vi "Main GNSS-Gmap.vi"() -> ()   [LabVIEW 2019]
uses:
  C:/Users/WEGO/Documents/GitHub/Ycar/LabVIEW/Gmap/dll/GMap.NET.WindowsForms.dll
  Gmap/dll/GMap.NET.WindowsForms.dll
  Ctrl/ublox-ui_main.ctl
  Ctrl/gnss_config-2.ctl
  Ctrl/cmd_RW.ctl
  Ctrl/cmd_ini-RW.ctl
  Ctrl/cmd_common.ctl
  Ctrl/comm-ini-rw-close.ctl
  Gmap/gmap_fgv-cmd.ctl
  Gmap/marker_info.ctl
panel:
  in  "main tap":enum32{"Main", "설정"}(tab)
  out "Ntrip conn":bool
  out "Sea Level":dbl
  out "N of Satellites":i32
  out "GNSS time":string
  in  "tm data reset":bool
  in  "gnss mode check":bool
  in  "GMapControl":refnum<k24>(container)
  out "TM graph":T1(graph)=[{"TM array"=[{"Y(E)"=195478.83340938148, "X(N)"=532749.6315443226}, {"Y(E)"=195478.83340938148, "X(N)"=532749.6315443226}, {"Y(E)"=195478.83340938148, "X(N)"=532749.6315443226}, {"Y(E)"=195478.83340938148, "X(N)"=532749.6315443226}, {"Y(E)"=195478.83340938148, "X(N)"=532749.6315443226}, {"Y(E)"=195478.83340938148, "X(N)"=532749.6315443226}, {"Y(E)"=195478.83340938148, "X(N)"=532749.6315443226}, {"Y(E)"=195478.83340938148, "X(N)"=532749.6315443226}, {"Y(E)"=195478.83340938148, "X(N)"=532749.6315443226}, {"Y(E)"=195478.83340938148, "X(N)"=532749.6315443226}, {"Y(E)"=195478.80387262133, "X(N)"=532749.5945652778}, {"Y(E)"=195478.80387262133, "X(N)"=532749.5945652778}, {"Y(E)"=195478.80387262133, "X(N)"=532749.5945652778}, {"Y(E)"=195478.80387262133, "X(N)"=532749.5945652778}, {"Y(E)"=195478.80387262133, "X(N)"=532749.5945652778}, {"Y(E)"=195478.80387262133, "X(N)"=532749.5945652778}, {"Y(E)"=195478.80387262133, "X(N)"=532749.5945652778}, {"Y(E)"=195478.80387262133, "X(N)"=532749.5945652778}, {"Y(E)"=195478.80387262133, "X(N)"=532749.5945652778}, {"Y(E)"=195478.80387262133, "X(N)"=532749.5945652778}, {"Y(E)"=195478.80387262133, "X(N)"=532749.5945652778}, {"Y(E)"=195478.80387262133, "X(N)"=532749.5945652778}, {"Y(E)"=195478.80387262133, "X(N)"=532749.5945652778}, {"Y(E)"=195478.86283602339, "X(N)"=532749.4650507653}, {"Y(E)"=195478.86283602339, "X(N)"=532749.4650507653}, {"Y(E)"=195478.86283602339, "X(N)"=532749.4650507653}, {"Y(E)"=195478.86283602339, "X(N)"=532749.4650507653}, {"Y(E)"=195478.86283602339, "X(N)"=532749.4650507653}, {"Y(E)"=195478.86283602339, "X(N)"=532749.4650507653}, {"Y(E)"=195478.86283602339, "X(N)"=532749.4650507653}, {"Y(E)"=195478.86283602339, "X(N)"=532749.4650507653}, {"Y(E)"=195478.86283602339, "X(N)"=532749.4650507653}, {"Y(E)"=195478.86283602339, "X(N)"=532749.4650507653}, {"Y(E)"=195478.86283602339, "X(N)"=532749.4650507653}, {"Y(E)"=195478.86283602339, "X(N)"=532749.4650507653}, {"Y(E)"=195478.86283602339, "X(N)"=532749.4650507653}, {"Y(E)"=195478.8185809412, "X(N)"=532749.5020697443}, {"Y(E)"=195478.8185809412, "X(N)"=532749.5020697443}, {"Y(E)"=195478.8185809412, "X(N)"=532749.5020697443}, {"Y(E)"=195478.8185809412, "X(N)"=532749.5020697443}, {"Y(E)"=195478.8185809412, "X(N)"=532749.5020697443}, {"Y(E)"=195478.8185809412, "X(N)"=532749.5020697443}, {"Y(E)"=195478.8185809412, "X(N)"=532749.5020697443}, {"Y(E)"=195478.8185809412, "X(N)"=532749.5020697443}, {"Y(E)"=195478.8185809412, "X(N)"=532749.5020697443}, {"Y(E)"=195478.8185809412, "X(N)"=532749.5020697443}, {"Y(E)"=195478.8185809412, "X(N)"=532749.5020697443}, {"Y(E)"=195478.8185809412, "X(N)"=532749.5020697443}, {"Y(E)"=195478.8185809412, "X(N)"=532749.5020697443}, {"Y(E)"=195478.8333493192, "X(N)"=532749.5205592669}, {"Y(E)"=195478.8333493192, "X(N)"=532749.5205592669}, {"Y(E)"=195478.8333493192, "X(N)"=532749.5205592669}, {"Y(E)"=195478.8333493192, "X(N)"=532749.5205592669}, {"Y(E)"=195478.8333493192, "X(N)"=532749.5205592669}, {"Y(E)"=195478.8333493192, "X(N)"=532749.5205592669}, {"Y(E)"=195478.8333493192, "X(N)"=532749.5205592669}, {"Y(E)"=195478.8333493192, "X(N)"=532749.5205592669}, {"Y(E)"=195478.8333493192, "X(N)"=532749.5205592669}, {"Y(E)"=195478.8333493192, "X(N)"=532749.5205592669}, {"Y(E)"=195478.8333493192, "X(N)"=532749.5205592669}, {"Y(E)"=195478.8333493192, "X(N)"=532749.5205592669}, {"Y(E)"=195478.81854089958, "X(N)"=532749.4280797082}, {"Y(E)"=195478.81854089958, "X(N)"=532749.4280797082}, {"Y(E)"=195478.81854089958, "X(N)"=532749.4280797082}, {"Y(E)"=195478.81854089958, "X(N)"=532749.4280797082}, {"Y(E)"=195478.81854089958, "X(N)"=532749.4280797082}, {"Y(E)"=195478.81854089958, "X(N)"=532749.4280797082}, {"Y(E)"=195478.81854089958, "X(N)"=532749.4280797082}, {"Y(E)"=195478.81854089958, "X(N)"=532749.4280797082}, {"Y(E)"=195478.81854089958, "X(N)"=532749.4280797082}, {"Y(E)"=195478.81854089958, "X(N)"=532749.4280797082}, {"Y(E)"=195478.81854089958, "X(N)"=532749.4280797082}, {"Y(E)"=195478.81854089958, "X(N)"=532749.4280797082}, {"Y(E)"=195478.81854089958, "X(N)"=532749.4280797082}, {"Y(E)"=195478.8332592258, "X(N)"=532749.3540816847}, {"Y(E)"=195478.8332592258, "X(N)"=532749.3540816847}, {"Y(E)"=195478.8332592258, "X(N)"=532749.3540816847}, {"Y(E)"=195478.8332592258, "X(N)"=532749.3540816847}, {"Y(E)"=195478.8332592258, "X(N)"=532749.3540816847}, {"Y(E)"=195478.8332592258, "X(N)"=532749.3540816847}, {"Y(E)"=195478.8332592258, "X(N)"=532749.3540816847}, {"Y(E)"=195478.8332592258, "X(N)"=532749.3540816847}, {"Y(E)"=195478.8332592258, "X(N)"=532749.3540816847}, {"Y(E)"=195478.8332592258, "X(N)"=532749.3540816847}, {"Y(E)"=195478.8332592258, "X(N)"=532749.3540816847}, {"Y(E)"=195478.8332592258, "X(N)"=532749.3540816847}, {"Y(E)"=195478.8332592258, "X(N)"=532749.3540816847}, {"Y(E)"=195478.61200383154, "X(N)"=532749.5761715989}, {"Y(E)"=195478.61200383154, "X(N)"=532749.5761715989}, {"Y(E)"=195478.61200383154, "X(N)"=532749.5761715989}, {"Y(E)"=195478.61200383154, "X(N)"=532749.5761715989}, {"Y(E)"=195478.61200383154, "X(N)"=532749.5761715989}, {"Y(E)"=195478.61200383154, "X(N)"=532749.5761715989}, {"Y(E)"=195478.61200383154, "X(N)"=532749.5761715989}, {"Y(E)"=195478.61200383154, "X(N)"=532749.5761715989}, {"Y(E)"=195478.61200383154, "X(N)"=532749.5761715989}, {"Y(E)"=195478.61200383154, "X(N)"=532749.5761715989}, {"Y(E)"=195478.61200383154, "X(N)"=532749.5761715989}, {"Y(E)"=195478.61200383154, "X(N)"=532749.5761715989}, {"Y(E)"=195478.61200383154, "X(N)"=532749.5761715989}, {"Y(E)"=195478.61197379892, "X(N)"=532749.5206790727}, {"Y(E)"=195478.61197379892, "X(N)"=532749.5206790727}, {"Y(E)"=195478.61197379892, "X(N)"=532749.5206790727}, {"Y(E)"=195478.61197379892, "X(N)"=532749.5206790727}, {"Y(E)"=195478.61197379892, "X(N)"=532749.5206790727}, {"Y(E)"=195478.61197379892, "X(N)"=532749.5206790727}, {"Y(E)"=195478.61197379892, "X(N)"=532749.5206790727}, {"Y(E)"=195478.61197379892, "X(N)"=532749.5206790727}, {"Y(E)"=195478.61197379892, "X(N)"=532749.5206790727}, {"Y(E)"=195478.61197379892, "X(N)"=532749.5206790727}, {"Y(E)"=195478.61197379892, "X(N)"=532749.5206790727}, {"Y(E)"=195478.61197379892, "X(N)"=532749.5206790727}, {"Y(E)"=195478.61197379892, "X(N)"=532749.5206790727}, {"Y(E)"=195478.64144048005, "X(N)"=532749.4281755526}, {"Y(E)"=195478.64144048005, "X(N)"=532749.4281755526}, {"Y(E)"=195478.64144048005, "X(N)"=532749.4281755526}, {"Y(E)"=195478.64144048005, "X(N)"=532749.4281755526}, {"Y(E)"=195478.64144048005, "X(N)"=532749.4281755526}, {"Y(E)"=195478.64144048005, "X(N)"=532749.4281755526}, {"Y(E)"=195478.64144048005, "X(N)"=532749.4281755526}, {"Y(E)"=195478.64144048005, "X(N)"=532749.4281755526}, {"Y(E)"=195478.64144048005, "X(N)"=532749.4281755526}, {"Y(E)"=195478.64144048005, "X(N)"=532749.4281755526}, {"Y(E)"=195478.64144048005, "X(N)"=532749.4281755526}, {"Y(E)"=195478.64144048005, "X(N)"=532749.4281755526}, {"Y(E)"=195478.64144048005, "X(N)"=532749.4281755526}, {"Y(E)"=195478.56754852948, "X(N)"=532749.2432403986}, {"Y(E)"=195478.56754852948, "X(N)"=532749.2432403986}, {"Y(E)"=195478.56754852948, "X(N)"=532749.2432403986}, {"Y(E)"=195478.56754852948, "X(N)"=532749.2432403986}, {"Y(E)"=195478.56754852948, "X(N)"=532749.2432403986}, {"Y(E)"=195478.56754852948, "X(N)"=532749.2432403986}, {"Y(E)"=195478.56754852948, "X(N)"=532749.2432403986}, {"Y(E)"=195478.56754852948, "X(N)"=532749.2432403986}, {"Y(E)"=195478.56754852948, "X(N)"=532749.2432403986}, {"Y(E)"=195478.56754852948, "X(N)"=532749.2432403986}, {"Y(E)"=195478.56754852948, "X(N)"=532749.2432403986}, {"Y(E)"=195478.56754852948, "X(N)"=532749.2432403986}, {"Y(E)"=195478.56754852948, "X(N)"=532749.2432403986}, {"Y(E)"=195478.5822568451, "X(N)"=532749.1507448669}, {"Y(E)"=195478.5822568451, "X(N)"=532749.1507448669}, {"Y(E)"=195478.5822568451, "X(N)"=532749.1507448669}, {"Y(E)"=195478.5822568451, "X(N)"=532749.1507448669}, {"Y(E)"=195478.5822568451, "X(N)"=532749.1507448669}, {"Y(E)"=195478.5822568451, "X(N)"=532749.1507448669}, {"Y(E)"=195478.5822568451, "X(N)"=532749.1507448669}, {"Y(E)"=195478.5822568451, "X(N)"=532749.1507448669}, {"Y(E)"=195478.5822568451, "X(N)"=532749.1507448669}, {"Y(E)"=195478.5822568451, "X(N)"=532749.1507448669}, {"Y(E)"=195478.5822568451, "X(N)"=532749.1507448669}, {"Y(E)"=195478.5822568451, "X(N)"=532749.1507448669}, {"Y(E)"=195478.5822568451, "X(N)"=532749.1507448669}, {"Y(E)"=195478.3755095352, "X(N)"=532748.9103890732}, {"Y(E)"=195478.3755095352, "X(N)"=532748.9103890732}, {"Y(E)"=195478.3755095352, "X(N)"=532748.9103890732}, {"Y(E)"=195478.3755095352, "X(N)"=532748.9103890732}, {"Y(E)"=195478.3755095352, "X(N)"=532748.9103890732}, {"Y(E)"=195478.3755095352, "X(N)"=532748.9103890732}, {"Y(E)"=195478.3755095352, "X(N)"=532748.9103890732}, {"Y(E)"=195478.3755095352, "X(N)"=532748.9103890732}, {"Y(E)"=195478.3755095352, "X(N)"=532748.9103890732}, {"Y(E)"=195478.3755095352, "X(N)"=532748.9103890732}, {"Y(E)"=195478.3755095352, "X(N)"=532748.9103890732}, {"Y(E)"=195478.3755095352, "X(N)"=532748.9103890732}, {"Y(E)"=195478.3755095352, "X(N)"=532748.9103890732}, {"Y(E)"=195478.37543945547, "X(N)"=532748.78090651}, {"Y(E)"=195478.37543945547, "X(N)"=532748.78090651}, {"Y(E)"=195478.37543945547, "X(N)"=532748.78090651}, {"Y(E)"=195478.37543945547, "X(N)"=532748.78090651}, {"Y(E)"=195478.37543945547, "X(N)"=532748.78090651}, {"Y(E)"=195478.37543945547, "X(N)"=532748.78090651}, {"Y(E)"=195478.37543945547, "X(N)"=532748.78090651}, {"Y(E)"=195478.37543945547, "X(N)"=532748.78090651}, {"Y(E)"=195478.37543945547, "X(N)"=532748.78090651}, {"Y(E)"=195478.37543945547, "X(N)"=532748.78090651}, {"Y(E)"=195478.37543945547, "X(N)"=532748.78090651}, {"Y(E)"=195478.37543945547, "X(N)"=532748.78090651}, {"Y(E)"=195478.5082848043, "X(N)"=532748.8178296402}, {"Y(E)"=195478.5082848043, "X(N)"=532748.8178296402}, {"Y(E)"=195478.5082848043, "X(N)"=532748.8178296402}, {"Y(E)"=195478.5082848043, "X(N)"=532748.8178296402}, {"Y(E)"=195478.5082848043, "X(N)"=532748.8178296402}, {"Y(E)"=195478.5082848043, "X(N)"=532748.8178296402}, {"Y(E)"=195478.5082848043, "X(N)"=532748.8178296402}, {"Y(E)"=195478.5082848043, "X(N)"=532748.8178296402}, {"Y(E)"=195478.5082848043, "X(N)"=532748.8178296402}, {"Y(E)"=195478.5082848043, "X(N)"=532748.8178296402}, {"Y(E)"=195478.5082848043, "X(N)"=532748.8178296402}, {"Y(E)"=195478.5082848043, "X(N)"=532748.8178296402}, {"Y(E)"=195478.5082848043, "X(N)"=532748.8178296402}, {"Y(E)"=195478.7001636224, "X(N)"=532748.8547208244}, {"Y(E)"=195478.7001636224, "X(N)"=532748.8547208244}, {"Y(E)"=195478.7001636224, "X(N)"=532748.8547208244}, {"Y(E)"=195478.7001636224, "X(N)"=532748.8547208244}, {"Y(E)"=195478.7001636224, "X(N)"=532748.8547208244}, {"Y(E)"=195478.7001636224, "X(N)"=532748.8547208244}, {"Y(E)"=195478.7001636224, "X(N)"=532748.8547208244}, {"Y(E)"=195478.7001636224, "X(N)"=532748.8547208244}, {"Y(E)"=195478.7001636224, "X(N)"=532748.8547208244}, {"Y(E)"=195478.7001636224, "X(N)"=532748.8547208244}]}, {"TM array"=[{"Y(E)"=195478.60442441847, "X(N)"=532749.6892681528}, {"Y(E)"=195478.63475492285, "X(N)"=532749.6883149784}, {"Y(E)"=195478.6649657266, "X(N)"=532749.6854592166}, {"Y(E)"=195478.69493760145, "X(N)"=532749.680712138}, {"Y(E)"=195478.72455226214, "X(N)"=532749.6740924771}, {"Y(E)"=195478.7536928331, "X(N)"=532749.6656263586}, {"Y(E)"=195478.7822443098, "X(N)"=532749.6553471944}, {"Y(E)"=195478.81009401265, "X(N)"=532749.6432955518}, {"Y(E)"=195478.83713203156, "X(N)"=532749.6295189931}, {"Y(E)"=195478.86325165984, "X(N)"=532749.6140718879}, {"Y(E)"=195478.88834981524, "X(N)"=532749.5970151991}, {"Y(E)"=195478.91232744683, "X(N)"=532749.5784162417}, {"Y(E)"=195478.93508992583, "X(N)"=532749.5583484169}, {"Y(E)"=195478.95654741913, "X(N)"=532749.5368909236}, {"Y(E)"=195478.97661524382, "X(N)"=532749.5141284446}, {"Y(E)"=195478.99521420136, "X(N)"=532749.490150813}, {"Y(E)"=195479.01227089018, "X(N)"=532749.4650526576}, {"Y(E)"=195479.02771799528, "X(N)"=532749.4389330294}, {"Y(E)"=195479.04149455403, "X(N)"=532749.4118950105}, {"Y(E)"=195479.0535461966, "X(N)"=532749.3840453076}, {"Y(E)"=195479.06382536073, "X(N)"=532749.3554938309}, {"Y(E)"=195479.0722914792, "X(N)"=532749.32635326}, {"Y(E)"=195479.07891114015, "X(N)"=532749.2967385993}, {"Y(E)"=195479.0836582188, "X(N)"=532749.2667667244}, {"Y(E)"=195479.08651398055, "X(N)"=532749.2365559207}, {"Y(E)"=195479.08746715504, "X(N)"=532749.2062254163}, {"Y(E)"=195479.08651398055, "X(N)"=532749.1758949119}, {"Y(E)"=195479.0836582188, "X(N)"=532749.1456841081}, {"Y(E)"=195479.07891114015, "X(N)"=532749.1157122332}, {"Y(E)"=195479.0722914792, "X(N)"=532749.0860975726}, {"Y(E)"=195479.06382536073, "X(N)"=532749.0569570017}, {"Y(E)"=195479.0535461966, "X(N)"=532749.0284055249}, {"Y(E)"=195479.04149455403, "X(N)"=532749.000555822}, {"Y(E)"=195479.02771799528, "X(N)"=532748.9735178031}, {"Y(E)"=195479.01227089018, "X(N)"=532748.9473981749}, {"Y(E)"=195478.99521420136, "X(N)"=532748.9223000195}, {"Y(E)"=195478.97661524382, "X(N)"=532748.898322388}, {"Y(E)"=195478.95654741913, "X(N)"=532748.8755599089}, {"Y(E)"=195478.93508992583, "X(N)"=532748.8541024156}, {"Y(E)"=195478.91232744683, "X(N)"=532748.8340345909}, {"Y(E)"=195478.88834981524, "X(N)"=532748.8154356334}, {"Y(E)"=195478.86325165984, "X(N)"=532748.7983789446}, {"Y(E)"=195478.83713203156, "X(N)"=532748.7829318395}, {"Y(E)"=195478.81009401265, "X(N)"=532748.7691552808}, {"Y(E)"=195478.7822443098, "X(N)"=532748.7571036381}, {"Y(E)"=195478.7536928331, "X(N)"=532748.746824474}, {"Y(E)"=195478.72455226214, "X(N)"=532748.7383583555}, {"Y(E)"=195478.69493760145, "X(N)"=532748.7317386946}, {"Y(E)"=195478.6649657266, "X(N)"=532748.726991616}, {"Y(E)"=195478.63475492285, "X(N)"=532748.7241358542}, {"Y(E)"=195478.60442441847, "X(N)"=532748.7231826797}, {"Y(E)"=195478.5740939141, "X(N)"=532748.7241358542}, {"Y(E)"=195478.54388311034, "X(N)"=532748.726991616}, {"Y(E)"=195478.5139112355, "X(N)"=532748.7317386946}, {"Y(E)"=195478.4842965748, "X(N)"=532748.7383583555}, {"Y(E)"=195478.45515600385, "X(N)"=532748.746824474}, {"Y(E)"=195478.42660452714, "X(N)"=532748.7571036381}, {"Y(E)"=195478.3987548243, "X(N)"=532748.7691552808}, {"Y(E)"=195478.37171680538, "X(N)"=532748.7829318395}, {"Y(E)"=195478.3455971771, "X(N)"=532748.7983789446}, {"Y(E)"=195478.3204990217, "X(N)"=532748.8154356334}, {"Y(E)"=195478.29652139012, "X(N)"=532748.8340345909}, {"Y(E)"=195478.27375891112, "X(N)"=532748.8541024156}, {"Y(E)"=195478.25230141782, "X(N)"=532748.8755599089}, {"Y(E)"=195478.23223359312, "X(N)"=532748.898322388}, {"Y(E)"=195478.21363463558, "X(N)"=532748.9223000195}, {"Y(E)"=195478.19657794677, "X(N)"=532748.9473981749}, {"Y(E)"=195478.18113084167, "X(N)"=532748.9735178031}, {"Y(E)"=195478.16735428292, "X(N)"=532749.000555822}, {"Y(E)"=195478.15530264034, "X(N)"=532749.0284055249}, {"Y(E)"=195478.14502347622, "X(N)"=532749.0569570017}, {"Y(E)"=195478.13655735774, "X(N)"=532749.0860975726}, {"Y(E)"=195478.1299376968, "X(N)"=532749.1157122332}, {"Y(E)"=195478.12519061816, "X(N)"=532749.1456841081}, {"Y(E)"=195478.1223348564, "X(N)"=532749.1758949119}, {"Y(E)"=195478.1213816819, "X(N)"=532749.2062254163}, {"Y(E)"=195478.1223348564, "X(N)"=532749.2365559207}, {"Y(E)"=195478.12519061816, "X(N)"=532749.2667667244}, {"Y(E)"=195478.1299376968, "X(N)"=532749.2967385993}, {"Y(E)"=195478.13655735774, "X(N)"=532749.32635326}, {"Y(E)"=195478.14502347622, "X(N)"=532749.3554938309}, {"Y(E)"=195478.15530264034, "X(N)"=532749.3840453076}, {"Y(E)"=195478.16735428292, "X(N)"=532749.4118950105}, {"Y(E)"=195478.18113084167, "X(N)"=532749.4389330294}, {"Y(E)"=195478.19657794677, "X(N)"=532749.4650526576}, {"Y(E)"=195478.21363463558, "X(N)"=532749.490150813}, {"Y(E)"=195478.23223359312, "X(N)"=532749.5141284446}, {"Y(E)"=195478.25230141782, "X(N)"=532749.5368909236}, {"Y(E)"=195478.27375891112, "X(N)"=532749.5583484169}, {"Y(E)"=195478.29652139012, "X(N)"=532749.5784162417}, {"Y(E)"=195478.3204990217, "X(N)"=532749.5970151991}, {"Y(E)"=195478.3455971771, "X(N)"=532749.6140718879}, {"Y(E)"=195478.37171680538, "X(N)"=532749.6295189931}, {"Y(E)"=195478.3987548243, "X(N)"=532749.6432955518}, {"Y(E)"=195478.42660452714, "X(N)"=532749.6553471944}, {"Y(E)"=195478.45515600385, "X(N)"=532749.6656263586}, {"Y(E)"=195478.4842965748, "X(N)"=532749.6740924771}, {"Y(E)"=195478.5139112355, "X(N)"=532749.680712138}, {"Y(E)"=195478.54388311034, "X(N)"=532749.6854592166}, {"Y(E)"=195478.5740939141, "X(N)"=532749.6883149784}, {"Y(E)"=195478.60442441847, "X(N)"=532749.6892681528}]}, {"TM array"=[{"Y(E)"=195478.60442441847, "X(N)"=532750.2062254163}, {"Y(E)"=195478.667214938, "X(N)"=532750.2042521447}, {"Y(E)"=195478.72975765204, "X(N)"=532750.1983401176}, {"Y(E)"=195478.79180573305, "X(N)"=532750.188512667}, {"Y(E)"=195478.85311430565, "X(N)"=532750.1748085774}, {"Y(E)"=195478.91344141285, "X(N)"=532750.1572819325}, {"Y(E)"=195478.97254897116, "X(N)"=532750.1360019022}, {"Y(E)"=195479.03020371005, "X(N)"=532750.1110524688}, {"Y(E)"=195479.08617809258, "X(N)"=532750.0825320963}, {"Y(E)"=195479.14025121345, "X(N)"=532750.0505533417}, {"Y(E)"=195479.19220967076, "X(N)"=532750.0152424106}, {"Y(E)"=195479.24184840822, "X(N)"=532749.9767386591}, {"Y(E)"=195479.2889715244, "X(N)"=532749.9351940437}, {"Y(E)"=195479.3333930459, "X(N)"=532749.8907725222}, {"Y(E)"=195479.37493766125, "X(N)"=532749.843649406}, {"Y(E)"=195479.41344141285, "X(N)"=532749.7940106685}, {"Y(E)"=195479.44875234397, "X(N)"=532749.7420522113}, {"Y(E)"=195479.4807310985, "X(N)"=532749.6879790904}, {"Y(E)"=195479.50925147094, "X(N)"=532749.6320047078}, {"Y(E)"=195479.53420090437, "X(N)"=532749.5743499689}, {"Y(E)"=195479.55548093477, "X(N)"=532749.5152424106}, {"Y(E)"=195479.5730075796, "X(N)"=532749.4549153034}, {"Y(E)"=195479.5867116692, "X(N)"=532749.3936067309}, {"Y(E)"=195479.59653911978, "X(N)"=532749.3315586499}, {"Y(E)"=195479.6024511469, "X(N)"=532749.2690159358}, {"Y(E)"=195479.60442441847, "X(N)"=532749.2062254163}, {"Y(E)"=195479.6024511469, "X(N)"=532749.1434348967}, {"Y(E)"=195479.59653911978, "X(N)"=532749.0808921827}, {"Y(E)"=195479.5867116692, "X(N)"=532749.0188441017}, {"Y(E)"=195479.5730075796, "X(N)"=532748.9575355292}, {"Y(E)"=195479.55548093477, "X(N)"=532748.897208422}, {"Y(E)"=195479.53420090437, "X(N)"=532748.8381008636}, {"Y(E)"=195479.50925147094, "X(N)"=532748.7804461247}, {"Y(E)"=195479.4807310985, "X(N)"=532748.7244717422}, {"Y(E)"=195479.44875234397, "X(N)"=532748.6703986212}, {"Y(E)"=195479.41344141285, "X(N)"=532748.618440164}, {"Y(E)"=195479.37493766125, "X(N)"=532748.5688014266}, {"Y(E)"=195479.3333930459, "X(N)"=532748.5216783104}, {"Y(E)"=195479.2889715244, "X(N)"=532748.4772567889}, {"Y(E)"=195479.24184840822, "X(N)"=532748.4357121735}, {"Y(E)"=195479.19220967076, "X(N)"=532748.397208422}, {"Y(E)"=195479.14025121345, "X(N)"=532748.3618974908}, {"Y(E)"=195479.08617809258, "X(N)"=532748.3299187362}, {"Y(E)"=195479.03020371005, "X(N)"=532748.3013983638}, {"Y(E)"=195478.97254897116, "X(N)"=532748.2764489304}, {"Y(E)"=195478.91344141285, "X(N)"=532748.2551689}, {"Y(E)"=195478.85311430565, "X(N)"=532748.2376422551}, {"Y(E)"=195478.79180573305, "X(N)"=532748.2239381656}, {"Y(E)"=195478.72975765204, "X(N)"=532748.214110715}, {"Y(E)"=195478.667214938, "X(N)"=532748.2081986879}, {"Y(E)"=195478.60442441847, "X(N)"=532748.2062254163}, {"Y(E)"=195478.54163389895, "X(N)"=532748.2081986879}, {"Y(E)"=195478.4790911849, "X(N)"=532748.214110715}, {"Y(E)"=195478.4170431039, "X(N)"=532748.2239381656}, {"Y(E)"=195478.3557345313, "X(N)"=532748.2376422551}, {"Y(E)"=195478.2954074241, "X(N)"=532748.2551689}, {"Y(E)"=195478.2362998658, "X(N)"=532748.2764489304}, {"Y(E)"=195478.1786451269, "X(N)"=532748.3013983638}, {"Y(E)"=195478.12267074437, "X(N)"=532748.3299187362}, {"Y(E)"=195478.0685976235, "X(N)"=532748.3618974908}, {"Y(E)"=195478.0166391662, "X(N)"=532748.397208422}, {"Y(E)"=195477.96700042873, "X(N)"=532748.4357121735}, {"Y(E)"=195477.91987731255, "X(N)"=532748.4772567889}, {"Y(E)"=195477.87545579104, "X(N)"=532748.5216783104}, {"Y(E)"=195477.8339111757, "X(N)"=532748.5688014266}, {"Y(E)"=195477.7954074241, "X(N)"=532748.618440164}, {"Y(E)"=195477.76009649297, "X(N)"=532748.6703986212}, {"Y(E)"=195477.72811773844, "X(N)"=532748.7244717422}, {"Y(E)"=195477.699597366, "X(N)"=532748.7804461247}, {"Y(E)"=195477.67464793258, "X(N)"=532748.8381008636}, {"Y(E)"=195477.65336790218, "X(N)"=532748.897208422}, {"Y(E)"=195477.63584125735, "X(N)"=532748.9575355292}, {"Y(E)"=195477.62213716775, "X(N)"=532749.0188441017}, {"Y(E)"=195477.61230971717, "X(N)"=532749.0808921827}, {"Y(E)"=195477.60639769005, "X(N)"=532749.1434348967}, {"Y(E)"=195477.60442441847, "X(N)"=532749.2062254163}, {"Y(E)"=195477.60639769005, "X(N)"=532749.2690159358}, {"Y(E)"=195477.61230971717, "X(N)"=532749.3315586499}, {"Y(E)"=195477.62213716775, "X(N)"=532749.3936067309}, {"Y(E)"=195477.63584125735, "X(N)"=532749.4549153034}, {"Y(E)"=195477.65336790218, "X(N)"=532749.5152424106}, {"Y(E)"=195477.67464793258, "X(N)"=532749.5743499689}, {"Y(E)"=195477.699597366, "X(N)"=532749.6320047078}, {"Y(E)"=195477.72811773844, "X(N)"=532749.6879790904}, {"Y(E)"=195477.76009649297, "X(N)"=532749.7420522113}, {"Y(E)"=195477.7954074241, "X(N)"=532749.7940106685}, {"Y(E)"=195477.8339111757, "X(N)"=532749.843649406}, {"Y(E)"=195477.87545579104, "X(N)"=532749.8907725222}, {"Y(E)"=195477.91987731255, "X(N)"=532749.9351940437}, {"Y(E)"=195477.96700042873, "X(N)"=532749.9767386591}, {"Y(E)"=195478.0166391662, "X(N)"=532750.0152424106}, {"Y(E)"=195478.0685976235, "X(N)"=532750.0505533417}, {"Y(E)"=195478.12267074437, "X(N)"=532750.0825320963}, {"Y(E)"=195478.1786451269, "X(N)"=532750.1110524688}, {"Y(E)"=195478.2362998658, "X(N)"=532750.1360019022}, {"Y(E)"=195478.2954074241, "X(N)"=532750.1572819325}, {"Y(E)"=195478.3557345313, "X(N)"=532750.1748085774}, {"Y(E)"=195478.4170431039, "X(N)"=532750.188512667}, {"Y(E)"=195478.4790911849, "X(N)"=532750.1983401176}, {"Y(E)"=195478.54163389895, "X(N)"=532750.2042521447}, {"Y(E)"=195478.60442441847, "X(N)"=532750.2062254163}]}, {"TM array"=[{"Y(E)"=195478.60442441847, "X(N)"=532751.2062254163}, {"Y(E)"=195478.73000545753, "X(N)"=532751.2022788732}, {"Y(E)"=195478.8550908856, "X(N)"=532751.1904548189}, {"Y(E)"=195478.97918704763, "X(N)"=532751.1707999178}, {"Y(E)"=195479.10180419282, "X(N)"=532751.1433917385}, {"Y(E)"=195479.22245840722, "X(N)"=532751.1083384489}, {"Y(E)"=195479.34067352384, "X(N)"=532751.0657783881}, {"Y(E)"=195479.4559830016, "X(N)"=532751.0158795213}, {"Y(E)"=195479.56793176668, "X(N)"=532750.9588387763}, {"Y(E)"=195479.67607800843, "X(N)"=532750.8948812673}, {"Y(E)"=195479.77999492307, "X(N)"=532750.824259405}, {"Y(E)"=195479.879272398, "X(N)"=532750.7472519018}, {"Y(E)"=195479.97351863034, "X(N)"=532750.6641626711}, {"Y(E)"=195480.0623616733, "X(N)"=532750.5753196281}, {"Y(E)"=195480.14545090403, "X(N)"=532750.4810733958}, {"Y(E)"=195480.22245840722, "X(N)"=532750.3817959209}, {"Y(E)"=195480.29308026948, "X(N)"=532750.2778790062}, {"Y(E)"=195480.35703777857, "X(N)"=532750.1697327645}, {"Y(E)"=195480.4140785234, "X(N)"=532750.0577839994}, {"Y(E)"=195480.46397739026, "X(N)"=532749.9424745217}, {"Y(E)"=195480.50653745106, "X(N)"=532749.824259405}, {"Y(E)"=195480.54159074073, "X(N)"=532749.7036051906}, {"Y(E)"=195480.56899891995, "X(N)"=532749.5809880454}, {"Y(E)"=195480.5886538211, "X(N)"=532749.4568918834}, {"Y(E)"=195480.60047787533, "X(N)"=532749.3318064554}, {"Y(E)"=195480.60442441847, "X(N)"=532749.2062254163}, {"Y(E)"=195480.60047787533, "X(N)"=532749.0806443772}, {"Y(E)"=195480.5886538211, "X(N)"=532748.9555589492}, {"Y(E)"=195480.56899891995, "X(N)"=532748.8314627871}, {"Y(E)"=195480.54159074073, "X(N)"=532748.7088456419}, {"Y(E)"=195480.50653745106, "X(N)"=532748.5881914275}, {"Y(E)"=195480.46397739026, "X(N)"=532748.4699763109}, {"Y(E)"=195480.4140785234, "X(N)"=532748.3546668332}, {"Y(E)"=195480.35703777857, "X(N)"=532748.2427180681}, {"Y(E)"=195480.29308026948, "X(N)"=532748.1345718263}, {"Y(E)"=195480.22245840722, "X(N)"=532748.0306549117}, {"Y(E)"=195480.14545090403, "X(N)"=532747.9313774367}, {"Y(E)"=195480.0623616733, "X(N)"=532747.8371312044}, {"Y(E)"=195479.97351863034, "X(N)"=532747.7482881615}, {"Y(E)"=195479.879272398, "X(N)"=532747.6651989308}, {"Y(E)"=195479.77999492307, "X(N)"=532747.5881914275}, {"Y(E)"=195479.67607800843, "X(N)"=532747.5175695652}, {"Y(E)"=195479.56793176668, "X(N)"=532747.4536120562}, {"Y(E)"=195479.4559830016, "X(N)"=532747.3965713113}, {"Y(E)"=195479.34067352384, "X(N)"=532747.3466724445}, {"Y(E)"=195479.22245840722, "X(N)"=532747.3041123836}, {"Y(E)"=195479.10180419282, "X(N)"=532747.269059094}, {"Y(E)"=195478.97918704763, "X(N)"=532747.2416509148}, {"Y(E)"=195478.8550908856, "X(N)"=532747.2219960137}, {"Y(E)"=195478.73000545753, "X(N)"=532747.2101719594}, {"Y(E)"=195478.60442441847, "X(N)"=532747.2062254163}, {"Y(E)"=195478.47884337942, "X(N)"=532747.2101719594}, {"Y(E)"=195478.35375795135, "X(N)"=532747.2219960137}, {"Y(E)"=195478.22966178932, "X(N)"=532747.2416509148}, {"Y(E)"=195478.10704464413, "X(N)"=532747.269059094}, {"Y(E)"=195477.98639042972, "X(N)"=532747.3041123836}, {"Y(E)"=195477.8681753131, "X(N)"=532747.3466724445}, {"Y(E)"=195477.75286583535, "X(N)"=532747.3965713113}, {"Y(E)"=195477.64091707027, "X(N)"=532747.4536120562}, {"Y(E)"=195477.53277082852, "X(N)"=532747.5175695652}, {"Y(E)"=195477.42885391388, "X(N)"=532747.5881914275}, {"Y(E)"=195477.32957643896, "X(N)"=532747.6651989308}, {"Y(E)"=195477.2353302066, "X(N)"=532747.7482881615}, {"Y(E)"=195477.14648716364, "X(N)"=532747.8371312044}, {"Y(E)"=195477.0633979329, "X(N)"=532747.9313774367}, {"Y(E)"=195476.98639042972, "X(N)"=532748.0306549117}, {"Y(E)"=195476.91576856747, "X(N)"=532748.1345718263}, {"Y(E)"=195476.85181105838, "X(N)"=532748.2427180681}, {"Y(E)"=195476.79477031354, "X(N)"=532748.3546668332}, {"Y(E)"=195476.7448714467, "X(N)"=532748.4699763109}, {"Y(E)"=195476.7023113859, "X(N)"=532748.5881914275}, {"Y(E)"=195476.66725809622, "X(N)"=532748.7088456419}, {"Y(E)"=195476.639849917, "X(N)"=532748.8314627871}, {"Y(E)"=195476.62019501586, "X(N)"=532748.9555589492}, {"Y(E)"=195476.60837096162, "X(N)"=532749.0806443772}, {"Y(E)"=195476.60442441847, "X(N)"=532749.2062254163}, {"Y(E)"=195476.60837096162, "X(N)"=532749.3318064554}, {"Y(E)"=195476.62019501586, "X(N)"=532749.4568918834}, {"Y(E)"=195476.639849917, "X(N)"=532749.5809880454}, {"Y(E)"=195476.66725809622, "X(N)"=532749.7036051906}, {"Y(E)"=195476.7023113859, "X(N)"=532749.824259405}, {"Y(E)"=195476.7448714467, "X(N)"=532749.9424745217}, {"Y(E)"=195476.79477031354, "X(N)"=532750.0577839994}, {"Y(E)"=195476.85181105838, "X(N)"=532750.1697327645}, {"Y(E)"=195476.91576856747, "X(N)"=532750.2778790062}, {"Y(E)"=195476.98639042972, "X(N)"=532750.3817959209}, {"Y(E)"=195477.0633979329, "X(N)"=532750.4810733958}, {"Y(E)"=195477.14648716364, "X(N)"=532750.5753196281}, {"Y(E)"=195477.2353302066, "X(N)"=532750.6641626711}, {"Y(E)"=195477.32957643896, "X(N)"=532750.7472519018}, {"Y(E)"=195477.42885391388, "X(N)"=532750.824259405}, {"Y(E)"=195477.53277082852, "X(N)"=532750.8948812673}, {"Y(E)"=195477.64091707027, "X(N)"=532750.9588387763}, {"Y(E)"=195477.75286583535, "X(N)"=532751.0158795213}, {"Y(E)"=195477.8681753131, "X(N)"=532751.0657783881}, {"Y(E)"=195477.98639042972, "X(N)"=532751.1083384489}, {"Y(E)"=195478.10704464413, "X(N)"=532751.1433917385}, {"Y(E)"=195478.22966178932, "X(N)"=532751.1707999178}, {"Y(E)"=195478.35375795135, "X(N)"=532751.1904548189}, {"Y(E)"=195478.47884337942, "X(N)"=532751.2022788732}, {"Y(E)"=195478.60442441847, "X(N)"=532751.2062254163}]}, {"TM array"=[{"Y(E)"=195478.60442441847, "X(N)"=532752.2062254163}, {"Y(E)"=195478.79279597706, "X(N)"=532752.2003056016}, {"Y(E)"=195478.98042411916, "X(N)"=532752.1825695202}, {"Y(E)"=195479.16656836224, "X(N)"=532752.1530871685}, {"Y(E)"=195479.35049407996, "X(N)"=532752.1119748997}, {"Y(E)"=195479.5314754016, "X(N)"=532752.0593949652}, {"Y(E)"=195479.70879807652, "X(N)"=532751.995554874}, {"Y(E)"=195479.88176229317, "X(N)"=532751.9207065736}, {"Y(E)"=195480.04968544078, "X(N)"=532751.8351454564}, {"Y(E)"=195480.2119048034, "X(N)"=532751.7392091928}, {"Y(E)"=195480.36778017535, "X(N)"=532751.6332763993}, {"Y(E)"=195480.51669638773, "X(N)"=532751.5177651446}, {"Y(E)"=195480.65806573626, "X(N)"=532751.3931312986}, {"Y(E)"=195480.79133030074, "X(N)"=532751.259866734}, {"Y(E)"=195480.9159641468, "X(N)"=532751.1184973855}, {"Y(E)"=195481.0314754016, "X(N)"=532750.9695811732}, {"Y(E)"=195481.13740819498, "X(N)"=532750.8137058013}, {"Y(E)"=195481.2333444586, "X(N)"=532750.6514864386}, {"Y(E)"=195481.31890557587, "X(N)"=532750.483563291}, {"Y(E)"=195481.39375387615, "X(N)"=532750.3105990743}, {"Y(E)"=195481.45759396735, "X(N)"=532750.1332763993}, {"Y(E)"=195481.51017390186, "X(N)"=532749.9522950777}, {"Y(E)"=195481.55128617067, "X(N)"=532749.76836936}, {"Y(E)"=195481.58076852243, "X(N)"=532749.582225117}, {"Y(E)"=195481.59850460375, "X(N)"=532749.3945969748}, {"Y(E)"=195481.60442441847, "X(N)"=532749.2062254163}, {"Y(E)"=195481.59850460375, "X(N)"=532749.0178538577}, {"Y(E)"=195481.58076852243, "X(N)"=532748.8302257155}, {"Y(E)"=195481.55128617067, "X(N)"=532748.6440814725}, {"Y(E)"=195481.51017390186, "X(N)"=532748.4601557548}, {"Y(E)"=195481.45759396735, "X(N)"=532748.2791744332}, {"Y(E)"=195481.39375387615, "X(N)"=532748.1018517582}, {"Y(E)"=195481.31890557587, "X(N)"=532747.9288875415}, {"Y(E)"=195481.2333444586, "X(N)"=532747.760964394}, {"Y(E)"=195481.13740819498, "X(N)"=532747.5987450313}, {"Y(E)"=195481.0314754016, "X(N)"=532747.4428696594}, {"Y(E)"=195480.9159641468, "X(N)"=532747.293953447}, {"Y(E)"=195480.79133030074, "X(N)"=532747.1525840985}, {"Y(E)"=195480.65806573626, "X(N)"=532747.019319534}, {"Y(E)"=195480.51669638773, "X(N)"=532746.894685688}, {"Y(E)"=195480.36778017535, "X(N)"=532746.7791744332}, {"Y(E)"=195480.2119048034, "X(N)"=532746.6732416397}, {"Y(E)"=195480.04968544078, "X(N)"=532746.5773053762}, {"Y(E)"=195479.88176229317, "X(N)"=532746.4917442589}, {"Y(E)"=195479.70879807652, "X(N)"=532746.4168959586}, {"Y(E)"=195479.5314754016, "X(N)"=532746.3530558674}, {"Y(E)"=195479.35049407996, "X(N)"=532746.3004759329}, {"Y(E)"=195479.16656836224, "X(N)"=532746.2593636641}, {"Y(E)"=195478.98042411916, "X(N)"=532746.2298813123}, {"Y(E)"=195478.79279597706, "X(N)"=532746.212145231}, {"Y(E)"=195478.60442441847, "X(N)"=532746.2062254163}, {"Y(E)"=195478.4160528599, "X(N)"=532746.212145231}, {"Y(E)"=195478.2284247178, "X(N)"=532746.2298813123}, {"Y(E)"=195478.0422804747, "X(N)"=532746.2593636641}, {"Y(E)"=195477.858354757, "X(N)"=532746.3004759329}, {"Y(E)"=195477.67737343535, "X(N)"=532746.3530558674}, {"Y(E)"=195477.50005076043, "X(N)"=532746.4168959586}, {"Y(E)"=195477.32708654378, "X(N)"=532746.4917442589}, {"Y(E)"=195477.15916339617, "X(N)"=532746.5773053762}, {"Y(E)"=195476.99694403354, "X(N)"=532746.6732416397}, {"Y(E)"=195476.8410686616, "X(N)"=532746.7791744332}, {"Y(E)"=195476.69215244922, "X(N)"=532746.894685688}, {"Y(E)"=195476.55078310068, "X(N)"=532747.019319534}, {"Y(E)"=195476.4175185362, "X(N)"=532747.1525840985}, {"Y(E)"=195476.29288469013, "X(N)"=532747.293953447}, {"Y(E)"=195476.17737343535, "X(N)"=532747.4428696594}, {"Y(E)"=195476.07144064197, "X(N)"=532747.5987450313}, {"Y(E)"=195475.97550437835, "X(N)"=532747.760964394}, {"Y(E)"=195475.88994326108, "X(N)"=532747.9288875415}, {"Y(E)"=195475.8150949608, "X(N)"=532748.1018517582}, {"Y(E)"=195475.7512548696, "X(N)"=532748.2791744332}, {"Y(E)"=195475.6986749351, "X(N)"=532748.4601557548}, {"Y(E)"=195475.65756266628, "X(N)"=532748.6440814725}, {"Y(E)"=195475.62808031452, "X(N)"=532748.8302257155}, {"Y(E)"=195475.6103442332, "X(N)"=532749.0178538577}, {"Y(E)"=195475.60442441847, "X(N)"=532749.2062254163}, {"Y(E)"=195475.6103442332, "X(N)"=532749.3945969748}, {"Y(E)"=195475.62808031452, "X(N)"=532749.582225117}, {"Y(E)"=195475.65756266628, "X(N)"=532749.76836936}, {"Y(E)"=195475.6986749351, "X(N)"=532749.9522950777}, {"Y(E)"=195475.7512548696, "X(N)"=532750.1332763993}, {"Y(E)"=195475.8150949608, "X(N)"=532750.3105990743}, {"Y(E)"=195475.88994326108, "X(N)"=532750.483563291}, {"Y(E)"=195475.97550437835, "X(N)"=532750.6514864386}, {"Y(E)"=195476.07144064197, "X(N)"=532750.8137058013}, {"Y(E)"=195476.17737343535, "X(N)"=532750.9695811732}, {"Y(E)"=195476.29288469013, "X(N)"=532751.1184973855}, {"Y(E)"=195476.4175185362, "X(N)"=532751.259866734}, {"Y(E)"=195476.55078310068, "X(N)"=532751.3931312986}, {"Y(E)"=195476.69215244922, "X(N)"=532751.5177651446}, {"Y(E)"=195476.8410686616, "X(N)"=532751.6332763993}, {"Y(E)"=195476.99694403354, "X(N)"=532751.7392091928}, {"Y(E)"=195477.15916339617, "X(N)"=532751.8351454564}, {"Y(E)"=195477.32708654378, "X(N)"=532751.9207065736}, {"Y(E)"=195477.50005076043, "X(N)"=532751.995554874}, {"Y(E)"=195477.67737343535, "X(N)"=532752.0593949652}, {"Y(E)"=195477.858354757, "X(N)"=532752.1119748997}, {"Y(E)"=195478.0422804747, "X(N)"=532752.1530871685}, {"Y(E)"=195478.2284247178, "X(N)"=532752.1825695202}, {"Y(E)"=195478.4160528599, "X(N)"=532752.2003056016}, {"Y(E)"=195478.60442441847, "X(N)"=532752.2062254163}]}]
  in  "stop":bool
  in  "zoom":dbl(slide) scale=3.0..20.0
  in  "gmap center":bool
  in  "PinDropMrkr":T2(ring)=enum."red_dot" caption="Pin Drop Marker"
  out "n":i32
  out "Arr-size":i32
  out "Min circle R":dbl format="%.2g"
  out "gnss info":T3 {"HDOP" scale=0.0..10.0; "PDOP" scale=0.0..10.0; "2D Acc.m" scale=0.0..10.0; "Latitude" format="%.9f"; "Longitude" format="%.9f"; "3D Acc.m" scale=0.0..10.0}
  in  "G Lon":dbl format="%.7f"
  in  "G Lat":dbl format="%.7f"
  out "Serial buffer":u32(graph)
  out "error out":errorcluster
  in  "gnss tm config":enum32{"UI", "GNSS config", "Ntrip client"}(tab)
  out "gnss mode cnt":u32[](array[numeric])
  in  "Sel tyep":T4(ring)=enum."$GPGGA"
  out "read_buffer":string
  out "read raw":string
  out "Histogram Graph":cluster{i32[], dbl[]}(graph)
  in  "GNSS cfg":T5={"Port"="COM10", "rate"=115200, "time offset"=9}
  in  "Ref R":dbl=1.0 format="%.2f"
  in  "arr limit":i32=200
  in  "dt":u32=20
  in  "Ntrip client info":T6={"id"="seoul", "pwd"="seoul", "ref pt"="YONS-RTCM32-M5", "address"="gnss.eseoul.go.kr", "port "=2101}
  out "Ntrip valid":string
  out "rtcm recv":string
  out "NMEA val":bool
  in  "Lon Dbclk":dbl format="%.11f"
  in  "Lat Dbclk":dbl format="%.11f"
  out "TM array":cluster{"Y(E)":dbl, "X(N)":dbl}[](array[cluster])
  out "ycenter_TM":dbl
  out "xcenter_TM":dbl
  # "GNSS/GPS Test Program"
  # "https://github.com/yunbum\nmade by ybbaek"
  # "GPS/GNSS Tester w Ntrip client/ Gmap"
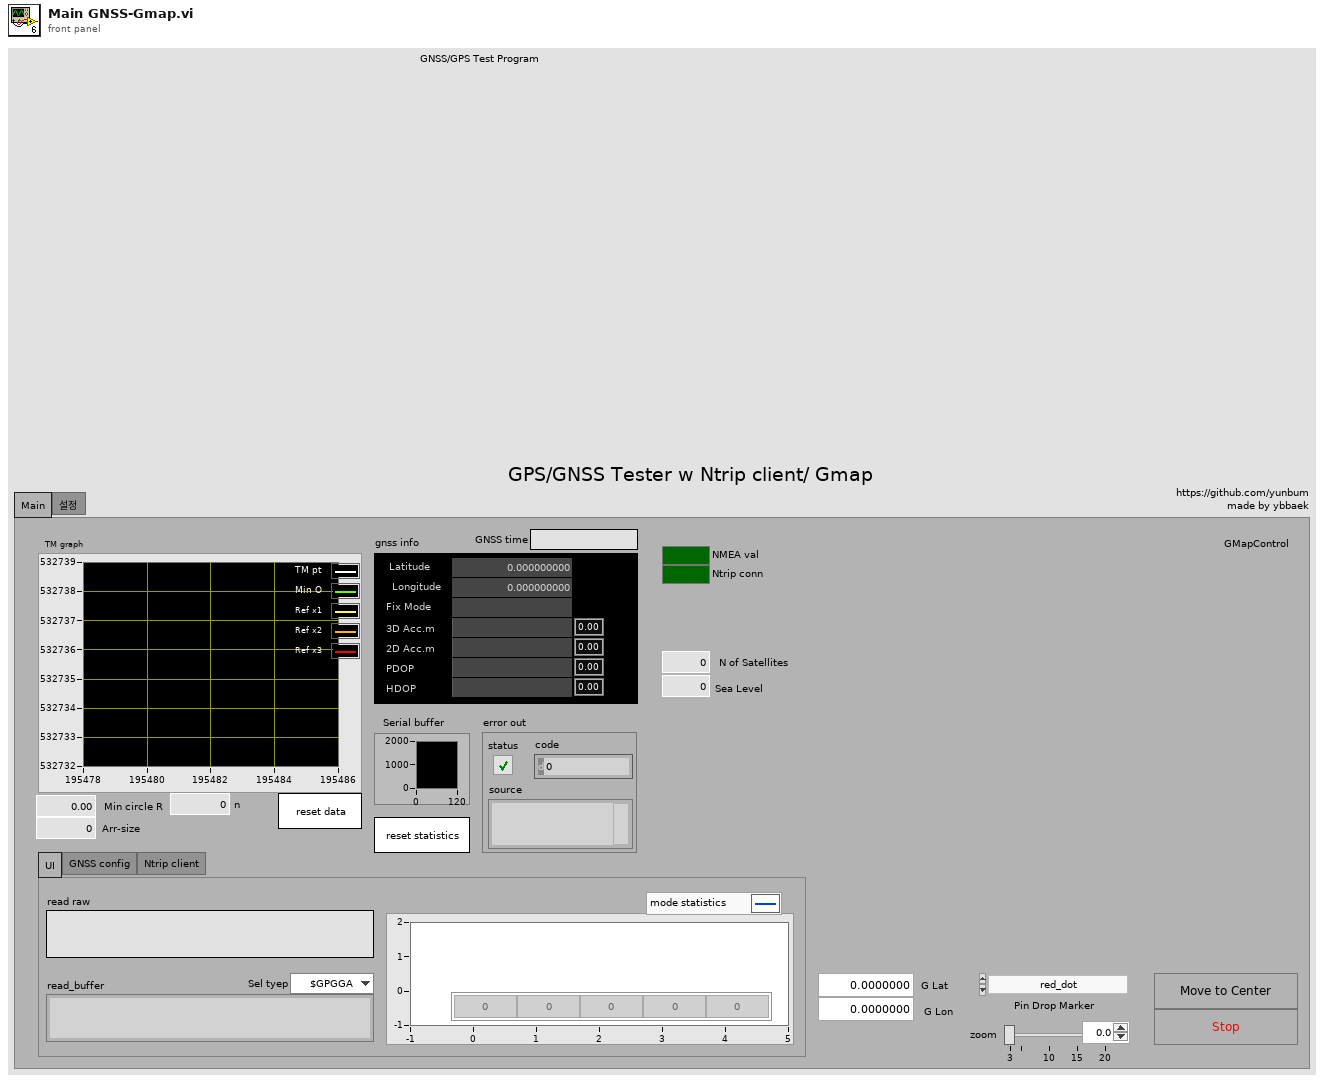
[diagram p1: front panel]
types:
  T1 = cluster{"TM array":cluster{"Y(E)":dbl, "X(N)":dbl}[]}[]
  T2 = enum16{"none", "arrow", "blue", "blue_small", "blue_dot", "blue_pushpin", "brown_small", "gray_small", "green", "green_small", "green_dot", "green_pushpin", "green_big_go", "yellow", "yellow_small", "yellow_dot", "yellow_big_pause", "yellow_pushpin", "lightblue", "lightblue_dot", "lightblue_pushpin", "orange", "orange_small", "orange_dot", "pink", "pink_dot", "pink_pushpin", "purple", "purple_small", "purple_dot", "purple_pushpin", "red", "red_small", "red_dot", "red_pushpin", "red_big_stop", "black_small", "white_small"}
  T3 = typedef "ublox-ui_main.ctl" = cluster{"Latitude":dbl, "Longitude":dbl, "Fix Mode":string, "3D Acc.m":dbl, "2D Acc.m":dbl, "PDOP":dbl, "HDOP":dbl}
  T4 = enum16{"$GPGSV", "$GLGSV", "$GPGGA", "$GAGSV", "$GBGSV", "$GNGLL", "$GNGGA", "$GNGSA", "$GNRMC", "$GNVTG"}
  T5 = typedef "gnss_config-2.ctl" = cluster{"Port":refnum<visa-resource-name>, "rate":u32, "time offset":u32}
  T6 = cluster{"id":string, "pwd":string, "ref pt":string, "address":string, "port ":u16}
  T7 = typedef "cmd_ini-RW.ctl" = enum16{"ini", "read", "write"}
  T8 = typedef "cmd_common.ctl" = enum16{"read", "write"}
  T9 = cluster{"G Lat":refnum<vi>, "G Lon":refnum<vi>, "Lat Dbclk":refnum<vi>, "Lon Dbclk":refnum<vi>, "zoom":refnum<vi>, "PinDropMrkr":refnum<vi>}
  T10 = typedef "comm-ini-rw-close.ctl" = enum16{"ini", "write", "read", "close"}
  T11 = typedef "gmap_fgv-cmd.ctl" = enum16{"marker type change", "save_image", "coll of points", "zoom n center markers", "add overlay reference", "read", "zoom", "set position by keyword", "set map provider", "map provider update", "create", "add marker", "clear marker", "close"}
  T12 = typedef "marker_info.ctl" = cluster{"arrLatLngActv":dbl[], "type":i32}
  T13 = cluster{"NA":u32, "valid":u32, "DGPS":u32, "RTK float":u32, "RTK fixed":u32}
  T14 = typedef "NMEA.lvlib/NMEA_LatitudeDirection.ctl" = enum16{"", "North", "South"}
  T15 = typedef "NMEA.lvlib/NMEA_LongitudeDirection.ctl" = enum16{"", "East", "West"}
  T16 = typedef "NMEA.lvlib/NMEA_GPS-Quality.ctl" = enum16{"Invalid", "GPS fix (SPS)", "DGPS fix", "PPS fix", "Real Time Kinematic", "Float RTK", "estimated", "Manual input mode", "Simulation mode"}
  T17 = cluster{"$GPGGA-message_OUT":cluster{"TimeStamp":timestamp, "Latitude":dbl, "Latitude-Direction":T14, "Longitude":dbl, "Longitude-Direction":T15, "GPS-Quality":T16, "N of Satellites":i32, "HDOP":dbl, "Altitude above Mean-Sea-Level":dbl, "Geoidal separation":dbl, "Time since last DGPS update":dbl, "DGPS reference station ID":i32}}
  T18 = cluster{"TM array":cluster{"Y(E)":dbl, "X(N)":dbl}[]}
  T19 = typedef "cmd_RW.ctl" = enum16{"read", "write"}
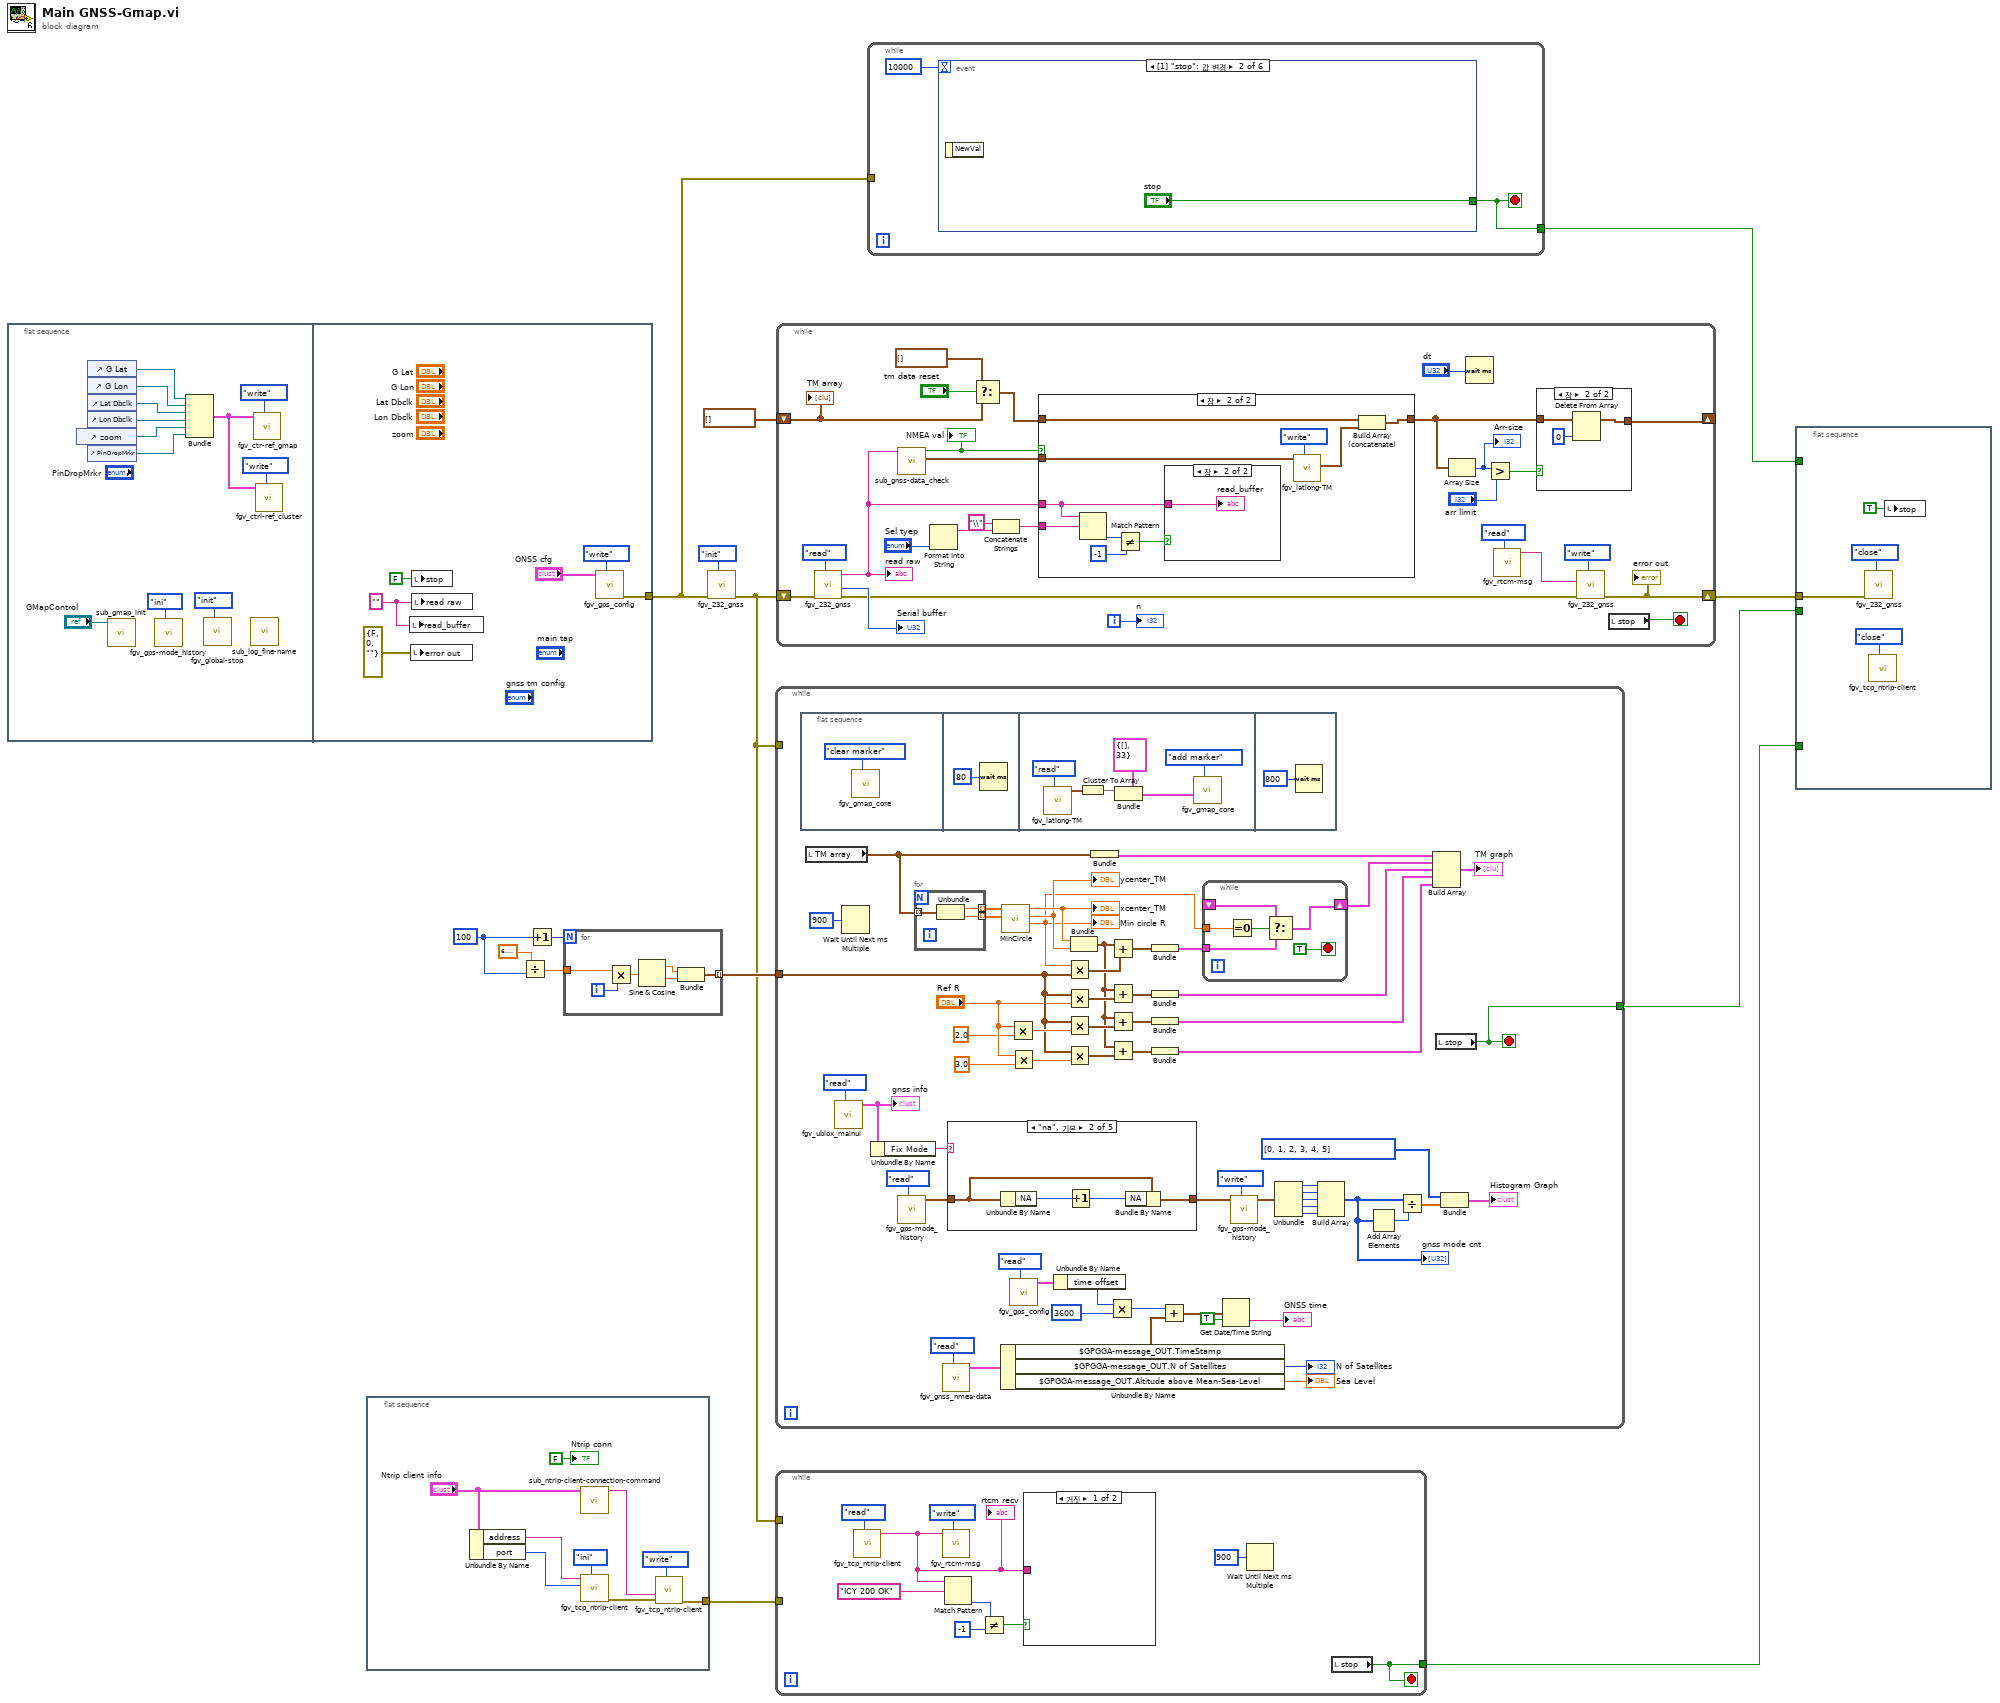
[diagram p0: block diagram]
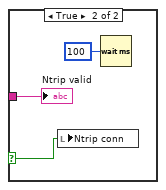
[diagram p2: hidden frame]
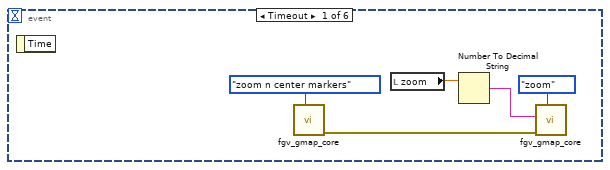
[diagram p3: hidden frame]
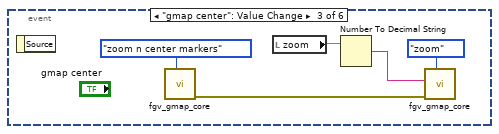
[diagram p4: hidden frame]
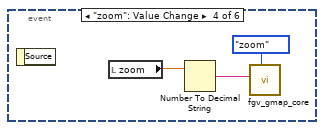
[diagram p5: hidden frame]
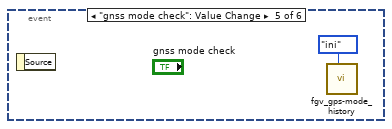
[diagram p6: hidden frame]
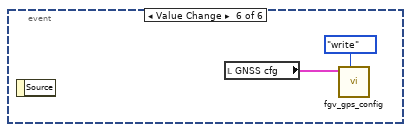
[diagram p7: hidden frame]
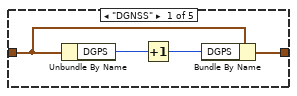
[diagram p8: hidden frame]
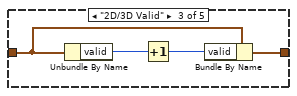
[diagram p9: hidden frame]
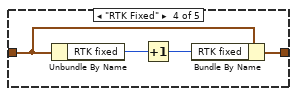
[diagram p10: hidden frame]
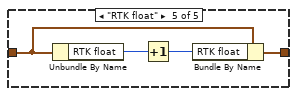
[diagram p11: hidden frame]
diagram:
  w8 = 100
  n1 = flat-sequence {
    tunnel: [w31] -> w11
    frame #0 {
      n2 = control-ref of="zoom"() -> (w20:refnum<vi>)
      n3 = control-ref of="G Lat"() -> (w24:refnum<vi>)
      n4 = control-ref of="G Lon"() -> (w23:refnum<vi>)
      n5 = control-ref of="Lat Dbclk"() -> (w22:refnum<vi>)
      n6 = control-ref of="Lon Dbclk"() -> (w21:refnum<vi>)
      n7 = control-ref of="PinDropMrkr"() -> (w19:refnum<vi>)
      n8 = call "sub_gmap_init.vi"("GMapControl"="GMapControl") -> ()  [unwired: 10 in, 1 out]
      n9 = call "fgv_gps-mode_history.vi"("cmd"=cmd_ini-RW."ini") -> ()  [unwired: 10 in, 1 out]
      n10 = Bundle("G Lat"=w24, "G Lon"=w23, "Lat Dbclk"=w22, "Lon Dbclk"=w21, "zoom"=w20, "PinDropMrkr"=w19) -> (w17:T9)  [unwired: 1 in]
      n11 = call "fgv_global-stop.vi"("cmd"=enum16{"init", "stop", "read"}."init") -> ()  [unwired: 10 in, 1 out]
      n12 = call "sub_log_fine-name.vi"() -> ()  [unwired: 11 in, 1 out]
      n13 = call "fgv_ctr-ref_gmap.vi"("cmd"=cmd_common."write", "ref in"=w17) -> ()  [unwired: 9 in, 1 out]
      n14 = call "fgv_ctrl-ref_cluster.vi"("cmd"=enum16{"read", "write"}."write", "ref"=w17) -> ()  [unwired: 9 in, 1 out]
    }
    frame #1 {
      w29 = "" ("read raw")
      n15 = local write "read_buffer"(w29) -> ()
      n16 = local write "error out"(errorcluster {"status"=FALSE, "code"=0, "source"=""} ("error out")) -> ()
      n17 = local write "stop"(FALSE ("정지")) -> ()
      n18 = local write "read raw"(w29) -> ()
      n19 = call "fgv_gps_config.vi"("cmd"=enum16{"read", "write"}."write", "GNSS cfg"="GNSS cfg") -> ("error out"=w31:errorcluster)  [unwired: 8 in, 1 out]
    }
  }
  n20 = flat-sequence {
    tunnel: [w38] -> w1
    frame #0 {
      n21 = Unbundle By Name("Ntrip client info") -> ("address"=w36:string, "port"=w35:u16)
      n22 = call "sub_ntrip-client-connection-command.vi"("Ntrip client info"="Ntrip client info") -> ("String"=w37:string)  [unwired: 10 in]
      n23 = call "fgv_tcp_ntrip-client.vi"("cmd"=comm-ini-rw-close."ini", "remote port"=w35, "address"=w36) -> ("error out"=w41:errorcluster)  [unwired: 7 in, 1 out]
      n24 = call "fgv_tcp_ntrip-client.vi"("cmd"=comm-ini-rw-close."write", "error in"=w41, "w-data"=w37) -> ("error out"=w38:errorcluster)  [unwired: 7 in, 1 out]
      "Ntrip conn" <- FALSE ("ntrip val")
    }
  }
  n25 = Divide(x=6.283185307179586, y=w8) -> (x/y=w9:dbl)
  n26 = Increment(x=w8) -> (x+1=w5:i32)
  n27 = for {
    N: w5 -> [_]
    tunnel: w9 -> [w46]
    tunnel: [w42] -> w6 mode=indexing
    i -> [w47]
    n28 = Multiply(x=w46, y=w47) -> (x*y=w45:dbl)
    n29 = Sine & Cosine(0:w45) -> (1:w44:dbl, 2:w43:dbl)
    n30 = Bundle(w44, w43) -> (w42:cluster{dbl, dbl})  [unwired: 1 in]
  }
  n31 = call "fgv_232_gnss.vi"("cmd"=enum16{"init", "read", "write", "close"}."init", "error in"=w11) -> ("error out"=w3:errorcluster)  [unwired: 7 in, 2 out]
  n32 = while {
    tunnel: w3 -> [_]
    tunnel: w6 -> [w70]
    tunnel: [w94] -> w4
    stop <- w94 stop-if-true
    n33 = flat-sequence {
      frame #0 {
        n34 = call "fgv_gmap_core.vi"("cmd"=gmap_fgv-cmd."clear marker") -> ()  [unwired: 7 in, 4 out]
      }
      frame #1 {
        n35 = Wait (ms)(milliseconds to wait=u32 80 ("대기 시간 (ms)")) -> ()  [unwired: 1 out]
      }
      frame #2 {
        n36 = call "fgv_latlong-TM.vi"("cmd"=enum16{"write", "read"}."read") -> ("latlong out"=w140:cluster{"lat":dbl, "long":dbl})  [unwired: 9 in, 1 out]
        n37 = Cluster To Array(cluster=w140) -> (array=w144:dbl[])
        n38 = Bundle(cluster=T12 {"arrLatLngActv"=[], "type"=33} ("marker_info"), "arrLatLngActv"=w144) -> (w142:T12)  [unwired: 1 in]
        n39 = call "fgv_gmap_core.vi"("cmd"=gmap_fgv-cmd."add marker", "marker_info"=w142) -> ()  [unwired: 6 in, 4 out]
      }
      frame #3 {
        n40 = Wait (ms)(milliseconds to wait=u32 800 ("대기 시간 (ms)")) -> ()  [unwired: 1 out]
      }
    }
    n41 = local read "TM array"() -> (w101:cluster{"Y(E)":dbl, "X(N)":dbl}[])
    n42 = call "fgv_ublox_mainui.vi"("cmd"=cmd_common."read") -> ("MainUI gnss out"=w93:T3)  [unwired: 10 in]
    "gnss info" <- w93
    n43 = Wait Until Next ms Multiple(millisecond multiple=u32 900 ("ms 배수")) -> ()  [unwired: 1 out]
    n44 = Unbundle By Name(w93) -> ("Fix Mode"=w92:string)
    n45 = call "fgv_gps-mode_history.vi"("cmd"=cmd_ini-RW."read") -> ("data out"=w89:T13)  [unwired: 10 in]
    n46 = for {
      tunnel: [w137] -> w107 mode=indexing
      tunnel: [w136] -> w106 mode=indexing
      tunnel: w101 -> [w135] mode=indexing
      n47 = Unbundle(w135) -> ("Y(E)"=w137:dbl, "X(N)"=w136:dbl)
    }
    n48 = call "fgv_gnss_nmea-data.vi"("cmd"=cmd_common."read") -> ("nmea-data out"=w53:T17)  [unwired: 10 in]
    n49 = case shown="\"na\", 기본" w92 {
      tunnel: w89 -> [w112 w116 w120 w124 w128]
      tunnel: [w111 w115 w119 w123 w127] -> w88
      frame "DGNSS" {
        n50 = Unbundle By Name(w112) -> ("DGPS"=w110:u32)
        n51 = Increment(x=w110) -> (x+1=w109:u32)
        n52 = Bundle By Name(cluster=w112, "DGPS"=w109) -> (w111:T13)
      }
      frame "na", Default {
        n53 = Unbundle By Name(w116) -> ("NA"=w114:u32)
        n54 = Increment(x=w114) -> (x+1=w113:u32)
        n55 = Bundle By Name(cluster=w116, "NA"=w113) -> (w115:T13)
      }
      frame "2D/3D Valid" {
        n56 = Unbundle By Name(w120) -> ("valid"=w118:u32)
        n57 = Increment(x=w118) -> (x+1=w117:u32)
        n58 = Bundle By Name(cluster=w120, "valid"=w117) -> (w119:T13)
      }
      frame "RTK Fixed" {
        n59 = Unbundle By Name(w124) -> ("RTK fixed"=w122:u32)
        n60 = Increment(x=w122) -> (x+1=w121:u32)
        n61 = Bundle By Name(cluster=w124, "RTK fixed"=w121) -> (w123:T13)
      }
      frame "RTK float" {
        n62 = Unbundle By Name(w128) -> ("RTK float"=w126:u32)
        n63 = Increment(x=w126) -> (x+1=w125:u32)
        n64 = Bundle By Name(cluster=w128, "RTK float"=w125) -> (w127:T13)
      }
    }
    n65 = Unbundle By Name(w53) -> ("$GPGGA-message_OUT.TimeStamp"=w52:timestamp, "$GPGGA-message_OUT.N of Satellites"=→"N of Satellites":i32, "$GPGGA-message_OUT.Altitude above Mean-Sea-Level"=→"Sea Level":dbl)
    n66 = call "MinCircle.vi"("y"=w106, "x"=w107) -> ("r"=w96:dbl, "yc"=w104:dbl, "xc"=w105:dbl)  [unwired: 6 in, 1 out]
    "xcenter_TM" <- w105
    "ycenter_TM" <- w104
    "Min circle R" <- w96
    n67 = Multiply(x="Ref R", y=2.0) -> (x*y=w73:dbl)
    n68 = Multiply(x="Ref R", y=3.0) -> (x*y=w72:dbl)
    n69 = call "fgv_gps_config.vi"("cmd"=enum16{"read", "write"}."read") -> ("GNSS cfg out"=w61:T5)  [unwired: 9 in, 1 out]
    n70 = Unbundle By Name(w61) -> ("time offset"=w60:u32)
    n71 = Multiply(x=w96, y=w70) -> (x*y=w103:cluster{dbl, dbl}[])
    n72 = Multiply(x=w70, y="Ref R") -> (x*y=w74:cluster{dbl, dbl}[])
    n73 = Multiply(x=w70, y=w73) -> (x*y=w75:cluster{dbl, dbl}[])
    n74 = Multiply(x=w70, y=w72) -> (x*y=w71:cluster{dbl, dbl}[])
    n75 = Bundle("xc"=w105, "yc"=w104) -> (w69:cluster{"xc":dbl, "yc":dbl})  [unwired: 1 in]
    n76 = Bundle("TM array"=w101) -> (w100:T18)  [unwired: 1 in]
    n77 = Multiply(x=w60, y=u32 3600) -> (x*y=w58:u32)
    n78 = Add(x=w69, y=w103) -> (x+y=w102:cluster{dbl, dbl}[])
    n79 = Add(x=w69, y=w74) -> (x+y=w77:cluster{dbl, dbl}[])
    n80 = Add(x=w69, y=w75) -> (x+y=w67:cluster{dbl, dbl}[])
    n81 = Add(x=w69, y=w71) -> (x+y=w68:cluster{dbl, dbl}[])
    n82 = Bundle(w102) -> (w98:cluster{cluster{dbl, dbl}[]})  [unwired: 1 in]
    n83 = Bundle(w77) -> (w76:cluster{cluster{dbl, dbl}[]})  [unwired: 1 in]
    n84 = Bundle(w67) -> (w66:cluster{cluster{dbl, dbl}[]})  [unwired: 1 in]
    n85 = Bundle(w68) -> (w65:cluster{cluster{dbl, dbl}[]})  [unwired: 1 in]
    n86 = Add(x=w58, y=w52) -> (x+y=w57:timestamp)
    n87 = while {
      shift-right: [w129] -> w97
      shift-left: _ -> [w131]
      tunnel: w96 -> [w133]
      tunnel: w98 -> [w130]
      stop <- TRUE stop-if-true
      n88 = Equal To 0?(x=w133) -> (x = 0?=w132:bool)
      n89 = Select(t=w131, s=w132, f=w130) -> (s? t:f=w129:cluster{cluster{dbl, dbl}[]})
    }
    n90 = Get Date/Time String(seconds (now)=w57, want seconds? (F)=TRUE ("초 보이기? (거짓)")) -> (time string=→"GNSS time":string)  [unwired: 1 in, 1 out]
    n91 = call "fgv_gps-mode_history.vi"("cmd"=cmd_ini-RW."write", "data"=w88) -> ("data out"=w87:T13)  [unwired: 9 in]
    n92 = Unbundle(w87) -> ("NA"=w86:u32, "valid"=w82:u32, "DGPS"=w83:u32, "RTK float"=w84:u32, "RTK fixed"=w85:u32)
    n93 = Build Array(w86, w82, w83, w84, w85) -> (w48:u32[])
    "gnss mode cnt" <- w48
    n94 = Add Array Elements(numeric array=w48) -> (sum=w79:u32)
    n95 = Divide(x=w48, y=w79) -> (x/y=w78:dbl[])
    n96 = Build Array(w100, w97, w76, w66, w65) -> (→"TM graph":T1)
    n97 = local read "stop"() -> (w94:bool)
    n98 = Bundle(i32[] [0, 1, 2, 3, 4, 5], w78) -> (→"Histogram Graph":cluster{i32[], dbl[]})  [unwired: 1 in]
  }
  n99 = while {
    tunnel: w3 -> [_]
    tunnel: [w154] -> w2
    tunnel: w1 -> [_]
    stop <- w154 stop-if-true
    n100 = call "fgv_tcp_ntrip-client.vi"("cmd"=comm-ini-rw-close."read") -> ("r-data"=w147:string)  [unwired: 9 in, 1 out]
    "rtcm recv" <- w147
    n101 = call "fgv_rtcm-msg.vi"("cmd"=cmd_RW."write", "rtcm msg"=w147) -> ()  [unwired: 9 in, 1 out]
    n102 = Match Pattern(string=w147, regular expression="ICY 200 OK" ("정규식")) -> (offset past match=w151:i32)  [unwired: 1 in, 3 out]
    n103 = Not Equal?(x=w151, y=-1) -> (x != y?=w148:bool)
    n104 = case shown="거짓" w148 {
      selector: w148 -> [_ w156]
      tunnel: w147 -> [_ w158]
      frame False {
      }
      frame True {
        n105 = local write "Ntrip conn"(w156) -> ()
        n106 = Wait (ms)(milliseconds to wait=u32 100 ("대기 시간 (ms)")) -> ()  [unwired: 1 out]
        "Ntrip valid" <- w158
      }
    }
    n107 = Wait Until Next ms Multiple(millisecond multiple=u32 900 ("ms 배수")) -> ()  [unwired: 1 out]
    n108 = local read "stop"() -> (w154:bool)
  }
  n109 = while {
    shift-right: [w173] -> _
    shift-left: cluster{"Y(E)":dbl, "X(N)":dbl}[] [] -> [w170]
    shift-right: [w159] -> w13
    shift-left: w3 -> [w183]
    i -> [w180]
    stop <- w164 stop-if-true
    n110 = call "fgv_232_gnss.vi"("cmd"=enum16{"init", "read", "write", "close"}."read", "error in"=w183) -> ("error out"=w162:errorcluster, "byte n"=→"Serial buffer":u32, "read_buffer"=w182:string)  [unwired: 7 in]
    "read raw" <- w182
    n111 = call "sub_gnss-data_check.vi"("gnss str"=w182) -> ("LatLong"=w179:cluster{dbl, dbl}, "val"=w178:bool)  [unwired: 8 in, 1 out]
    "NMEA val" <- w178
    n112 = Format Into String("Sel tyep") -> (resulting string=w167:string)  [unwired: 3 in, 1 out]
    n113 = Select(t=cluster{"Y(E)":dbl, "X(N)":dbl}[] [], s="tm data reset", f=w170) -> (s? t:f=w169:cluster{"Y(E)":dbl, "X(N)":dbl}[])
    n114 = Concatenate Strings("\\" ("string"), w167) -> (w165:string)
    n115 = case shown="참" w178 {
      tunnel: [w190 w200] -> w174
      tunnel: w169 -> [w190 w199]
      tunnel: w182 -> [_ w191]
      tunnel: w179 -> [_ w197]
      tunnel: w165 -> [_ w195]
      frame False {
      }
      frame True {
        n116 = Match Pattern(string=w191, regular expression=w195) -> (offset past match=w194:i32)  [unwired: 1 in, 3 out]
        n117 = Not Equal?(x=w194, y=-1) -> (x != y?=w192:bool)
        n118 = case shown="참" w192 {
          tunnel: w191 -> [_ w201]
          frame False {
          }
          frame True {
            "read_buffer" <- w201
          }
        }
        n119 = call "fgv_latlong-TM.vi"("cmd"=enum16{"write", "read"}."write", "latlong"=w197) -> ("tm out"=w196:cluster{"YE":dbl, "XN":dbl})  [unwired: 8 in, 1 out]
        n120 = Build Array (concatenate)(w199, w196) -> (w200:cluster{"YE":dbl, "XN":dbl}[])
      }
    }
    n121 = Array Size(array=w174) -> (size(s)=w177:i32)
    "Arr-size" <- w177
    n122 = Wait (ms)(milliseconds to wait="dt") -> ()  [unwired: 1 out]
    n123 = Greater?(x=w177, y="arr limit") -> (0:w175:bool)
    n124 = call "fgv_rtcm-msg.vi"("cmd"=cmd_RW."read") -> ("rtcm msg out"=w160:string)  [unwired: 10 in]
    n125 = case shown="참" w175 {
      tunnel: w174 -> [w186 w188]
      tunnel: [w186 w187] -> w173
      frame False {
      }
      frame True {
        n126 = Delete From Array(array=w188, index=0) -> (array with subset deleted=w187:cluster{"YE":dbl, "XN":dbl}[])  [unwired: 1 in, 1 out]
      }
    }
    n127 = call "fgv_232_gnss.vi"("cmd"=enum16{"init", "read", "write", "close"}."write", "error in"=w162, "write buff"=w160) -> ("error out"=w159:errorcluster)  [unwired: 6 in, 2 out]
    "error out" <- w159
    n128 = local read "stop"() -> (w164:bool)
    "n" <- w180
    "TM array" <- w170
  }
  n129 = while {
    tunnel: w11 -> [_]
    tunnel: [w203] -> w10
    stop <- w203 stop-if-true
    n130 = event shown="[1] \"stop\": 값 변경" {
      selector: _ -> [_ _ _ _ _ _]
      dyn-events: _ -> [_ _ _ _ _ _]
      timeout: 10000 -> [_ _ _ _ _ _]
      tunnel: [_ "stop" _ _ _ _] -> w203
      event Timeout {
        n131 = event-data() -> ()  [unwired: 1 in, 1 out]
        n132 = call "fgv_gmap_core.vi"("cmd"=gmap_fgv-cmd."zoom n center markers") -> ("error out"=w204:errorcluster)  [unwired: 7 in, 3 out]
        n133 = local read "zoom"() -> (w208:dbl)
        n134 = Number To Decimal String(number=w208) -> (decimal integer string=w207:string)  [unwired: 1 in]
        n135 = call "fgv_gmap_core.vi"(7:"cmd"=gmap_fgv-cmd."zoom" ("cmd"), "error in"=w204, 10:"cmd"=w207) -> ()  [unwired: 5 in, 4 out]
      }
      event "stop": Value Change {
        n136 = event-data() -> ()  [unwired: 1 in, 1 out]
      }
      event "gmap center": Value Change {
        n137 = event-data() -> ()  [unwired: 1 in, 1 out]
        n138 = call "fgv_gmap_core.vi"("cmd"=gmap_fgv-cmd."zoom n center markers") -> ("error out"=w210:errorcluster)  [unwired: 7 in, 3 out]
        n139 = local read "zoom"() -> (w213:dbl)
        n140 = Number To Decimal String(number=w213) -> (decimal integer string=w212:string)  [unwired: 1 in]
        n141 = call "fgv_gmap_core.vi"(7:"cmd"=gmap_fgv-cmd."zoom" ("cmd"), "error in"=w210, 10:"cmd"=w212) -> ()  [unwired: 5 in, 4 out]
      }
      event "zoom": Value Change {
        n142 = event-data() -> ()  [unwired: 1 in, 1 out]
        n143 = local read "zoom"() -> (w216:dbl)
        n144 = Number To Decimal String(number=w216) -> (decimal integer string=w215:string)  [unwired: 1 in]
        n145 = call "fgv_gmap_core.vi"(7:"cmd"=gmap_fgv-cmd."zoom" ("cmd"), 10:"cmd"=w215) -> ()  [unwired: 6 in, 4 out]
      }
      event "gnss mode check": Value Change {
        n146 = event-data() -> ()  [unwired: 1 in, 1 out]
        n147 = call "fgv_gps-mode_history.vi"("cmd"=cmd_ini-RW."ini") -> ()  [unwired: 10 in, 1 out]
      }
      event Value Change {
        n148 = event-data() -> ()  [unwired: 1 in, 1 out]
        n149 = local read "GNSS cfg"() -> (w219:T5)
        n150 = call "fgv_gps_config.vi"("cmd"=enum16{"read", "write"}."write", "GNSS cfg"=w219) -> ()  [unwired: 8 in, 2 out]
      }
    }
  }
  n151 = flat-sequence {
    tunnel: w13 -> [w223]
    tunnel: w4 -> [_]
    tunnel: w10 -> [_]
    tunnel: w2 -> [_]
    frame #0 {
      n152 = call "fgv_232_gnss.vi"("cmd"=enum16{"init", "read", "write", "close"}."close", "error in"=w223) -> ()  [unwired: 7 in, 3 out]
      n153 = call "fgv_tcp_ntrip-client.vi"("cmd"=comm-ini-rw-close."close") -> ()  [unwired: 9 in, 2 out]
      n154 = local write "stop"(TRUE ("stop")) -> ()
    }
  }
